vi "PublishHistory.vi"(8 "error in (no error)":errorcluster, 9 "Body":T1, 10 "Qbus in":refnum<class "Qbus.lvclass">, 11 "config in":T2) -> (0 "error out":errorcluster, 3 "config out":T2)   [LabVIEW 2017, in "TestPanel.lvlib"]
uses:
  <vilib>/addons/InsightCM/Devices/Shared/Common/TestPanel/TestPanel.lvlib
  <vilib>/addons/InsightCM/Devices/Shared/Common/TestPanel/controls/Configuration.ctl
  <vilib>/addons/InsightCM/Devices/Shared/Common/TestPanel/controls/State.ctl
  <vilib>/addons/InsightCM/MessageBus/Base/controls/IRoutingSource.ctl
  <vilib>/addons/Qbus/Qbus.lvclass
  <vilib>/addons/InsightCM/MessageBus/MessageLibrary/Device/controls/DeviceTestPanelGetTimeSeriesRequestBody.ctl
  <vilib>/addons/InsightCM/MessageBus/MessageLibrary/Device/controls/DeviceTestPanelGetTimeSeriesResponseBody.ctl
  <vilib>/addons/InsightCM/MessageBus/Base/controls/TestPanelHistory.ctl
  <vilib>/addons/InsightCM/MessageBus/Base/controls/KeyValuePair.ctl
  <vilib>/addons/InsightCM/MessageBus/Base/controls/TestPanelTimeSeries.ctl
  <vilib>/addons/InsightCM/MessageBus/Base/controls/TestPanelValue.ctl
  <vilib>/addons/InsightCM/Devices/Shared/Common/ServerComm/ServerComm.lvlib
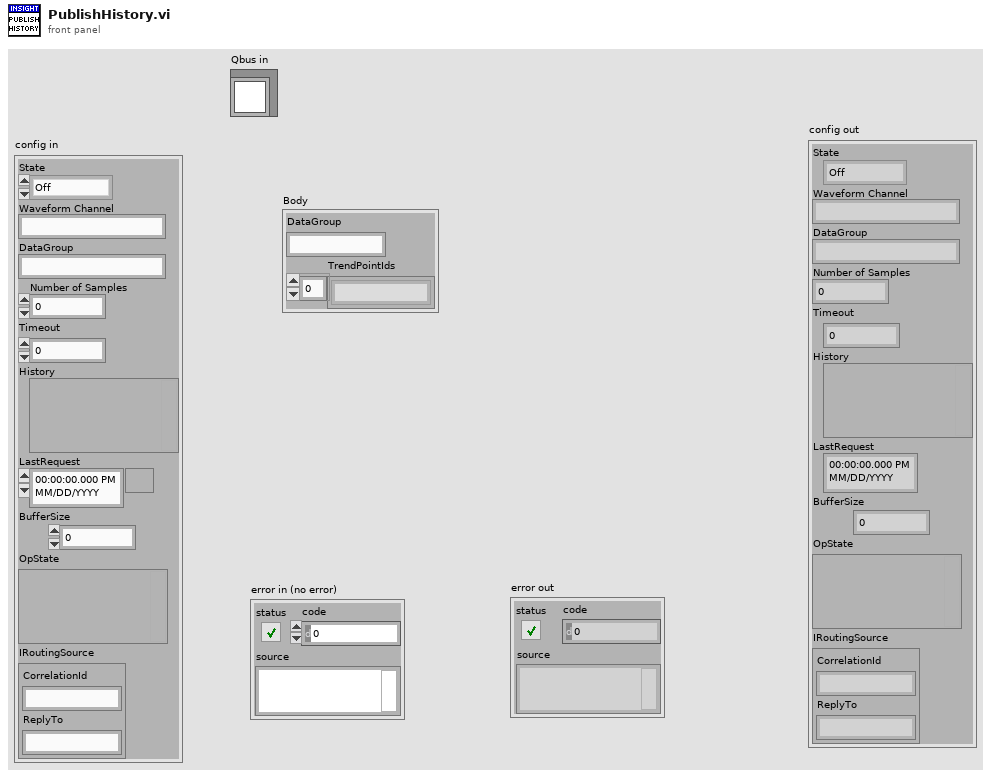
[diagram p1: front panel]
types:
  T1 = typedef "DeviceTestPanelGetTimeSeriesRequestBody.ctl" = cluster{"DataGroup":string, "TrendPointIds":string[]}
  T2 = typedef "TestPanel.lvlib/Configuration.ctl" = cluster{"State":T3, "Waveform Channel":string, "DataGroup":string, "Number of Samples":i32, "Timeout":dbl, "History":variant, "LastRequest":timestamp, "BufferSize":i32, "OpState":variant, "IRoutingSource":T4}
  T3 = typedef "TestPanel.lvlib/State.ctl" = enum16{"Off", "On", "PendingValues", "PendingDataSet"}
  T4 = typedef "IRoutingSource.ctl" = cluster{"CorrelationId":string, "ReplyTo":string}
  T5 = typedef "DeviceTestPanelGetTimeSeriesResponseBody.ctl" = cluster{"Data":T6}
  T6 = typedef "TestPanelHistory.ctl" = cluster{"DataGroup":string, "OperatingState":string, "ChannelStatus":T7[], "TimeSeries":T8[]}
  T7 = typedef "KeyValuePair.ctl" = cluster{"Key":string, "Value":string}
  T8 = typedef "TestPanelTimeSeries.ctl" = cluster{"TrendPointId":string, "AssetName":string, "MetricName":string, "Unit":string, "Values":T9[]}
  T9 = typedef "TestPanelValue.ctl" = cluster{"Value":dbl, "Timestamp":i64, "Invalid":bool}
  T10 = typedef "Message.ctl" = cluster{"Header":T11, "Body":u8[]}
  T11 = typedef "MessageHeader.ctl" = cluster{"MessageName":string, "Timestamp":i64, "CorrelationId":string, "ContentType":string, "RoutingKey":string, "Properties":T7[]}
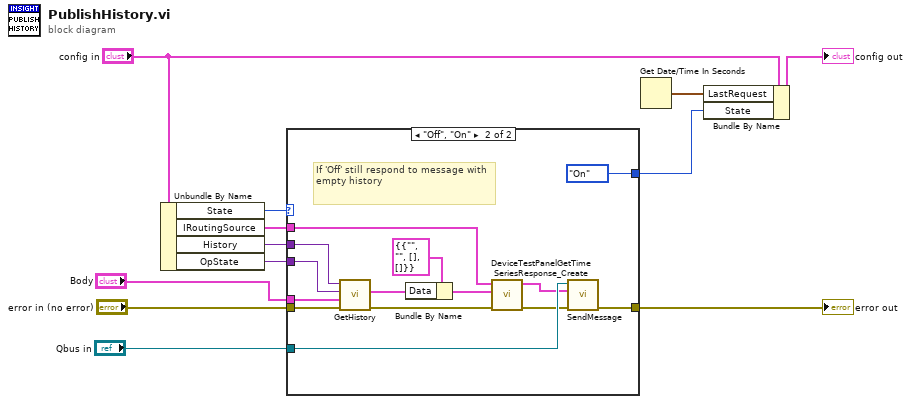
[diagram p0: block diagram]
diagram:
  n1 = Unbundle By Name("config in") -> ("State"=w9:T3, "IRoutingSource"=w5:T4, "History"=w8:variant, "OpState"=w7:variant)
  n2 = case shown="\"Off\", \"On\"" w9 {
    selector: w9 -> [w14 _]
    tunnel: w8 -> [_ w25]
    tunnel: w7 -> [_ w26]
    tunnel: "error in (no error)" -> [w13 w24]
    tunnel: w5 -> [_ w19]
    tunnel: "Qbus in" -> [_ w28]
    tunnel: [w13 w27] -> w3
    tunnel: [w14 State."On" ("State")] -> w2
    tunnel: "Body" -> [_ w16]
    frame "PendingValues", "PendingDataSet" {
    }
    frame "Off", "On" {
      # "If 'Off' still respond to message with empty history"
      n3 = call <vilib>:"GetHistory.vi"("error in (no error)"=w24, "Body"=w16, "OpState"=w26, "History"=w25) -> ("error out"=w22:errorcluster, "time series"=w17:T6)  [unwired: 6 in]
      n4 = Bundle By Name(cluster=T5 {"Data"={"DataGroup"="", "OperatingState"="", "ChannelStatus"=[], "TimeSeries"=[]}} ("DeviceTestPanelGetTimeSeriesResponse"), "Data"=w17) -> (w20:T5)
      n5 = call <vilib>:"DeviceTestPanelGetTimeSeriesResponse_Create.vi"("error in (no error)"=w22, "DeviceTestPanelGetTimeSeriesResponse"=w20, "IRoutingSource"=w19) -> ("error out"=w23:errorcluster, "Message"=w18:T10)  [unwired: 7 in]
      n6 = call <vilib>:"SendMessage.vi"("error in (no error)"=w23, "message"=w18, "Qbus in"=w28) -> ("error out"=w27:errorcluster)  [unwired: 7 in, 1 out]
    }
  }
  "error out" <- w3
  n7 = Get Date/Time In Seconds() -> (seconds since 1Jan1904=w10:timestamp)
  n8 = Bundle By Name(cluster="config in", "LastRequest"=w10, "State"=w2) -> (→"config out":T2)
